vi "Pre Launch Init.vi"(11 "UI in":refnum<class "UI.lvclass"> caption="操作者输入") -> (0 "error out":errorcluster caption="错误输出", 3 "UI out":refnum<class "UI.lvclass"> caption="操作者输出")   [LabVIEW 2019, in "UI.lvlib" / "UI.lvclass"]
doc: "(<B>文件名</B>: Actor Framework.lvlib:Actor.lvclass:Pre Launch Init.vi)\n\n定义启动嵌套操作者方法被调用之后、操作者核心方法开始运行之前的操作。\n\n默认情况下，该方法不执行任何操作。子孙类重写该方法定义具体的操作。"
uses:
  UI.lvclass
  C:/Program Files (x86)/National Instruments/LabVIEW 2019/vi.lib/ActorFramework/Actor/Actor.lvclass
  <vilib>/ActorFramework/Actor/Actor.lvclass/Actor.ctl
  <vilib>/ActorFramework/Message Enqueuer/Message Enqueuer.lvclass/Message Enqueuer.ctl
  <vilib>/ActorFramework/Message Enqueuer/Enqueue.vi
  <vilib>/ActorFramework/Message Enqueuer/Init from Existing Queue.vi
  C:/Program Files (x86)/National Instruments/LabVIEW 2019/vi.lib/ActorFramework/Message/Message.lvclass
  <vilib>/ActorFramework/Message Priority Queue/Priority Enqueue.vi
  <vilib>/ActorFramework/Message Enqueuer/Message Enqueuer.lvclass
  <vilib>/ActorFramework/Actor/Actor.lvclass
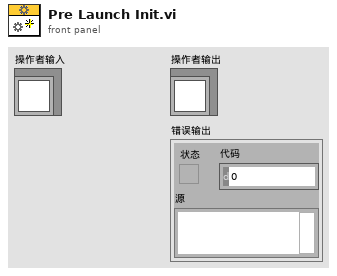
[diagram p1: front panel]
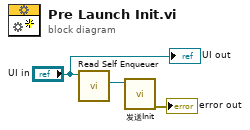
[diagram p0: block diagram]
diagram:
  n1 = call <vilib>:"Read Self Enqueuer.vi"("Actor"="UI in") -> ("Self Enqueuer"=w1:refnum<class "Message Enqueuer.lvclass">)  [unwired: 10 in]
  n2 = call "发送Init.vi"("Message Enqueuer"=w1) -> ("error out"=→"error out":errorcluster)  [unwired: 9 in, 1 out]
  "UI out" <- "UI in"
